vi "Y.vi"(8 "error in (no error)":errorcluster, 11 "MagSpec_Bella in":refnum<class "MagSpec_Bella.lvclass">) -> (0 "error out":errorcluster, 3 "MagSpec_Bella out":refnum<class "MagSpec_Bella.lvclass">)   [LabVIEW 2013, in "MagSpec_Bella.lvclass"]
uses:
  MagSpec_Bella.lvclass
  Controls/finalCalib--Cluster.ctl
  MagSpec_Bella.lvclass/MagSpec_Bella.ctl
  <vilib>/Analysis/1siggen.llb/Ramp Pattern by Delta.vi
  <vilib>/Analysis/NI_AALBase.lvlib
panel:
  out "Working":i32[](array[numeric])
  out "GOOD - not working":i32[](array[numeric])
  out "G":i32[](array[numeric])
  out "pixel angle (y)(pixel)":dbl[][](graph)
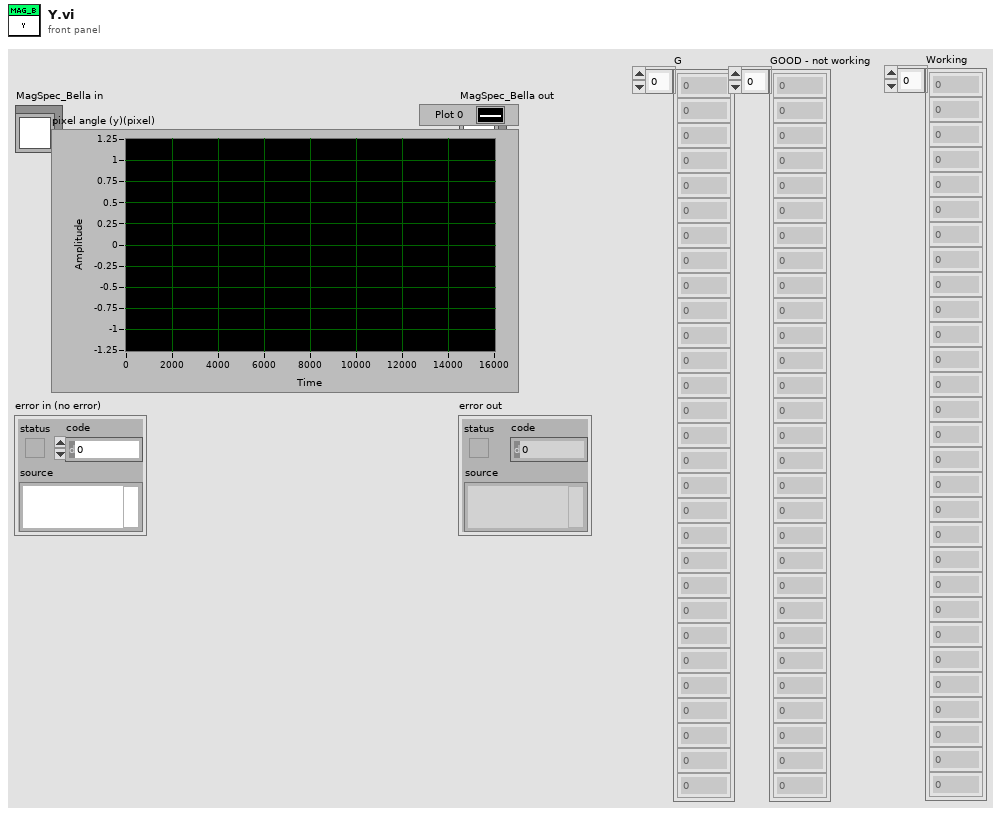
[diagram p1: front panel]
types:
  T1 = typedef "finalCalib--Cluster.ctl" = cluster{"X":dbl[][], "xi":dbl[][], "delta momentum":dbl, "Y":dbl[][], "yi":dbl[][], "angle (Y)":dbl[], "delta angle":dbl, "scale delta angle":dbl, "intraX":dbl, "intraY":dbl, "mask":dbl[][]}
  T2 = typedef "Calibration_Pixel_based.ctl" = cluster{"y1(pixel)":dbl[], "y2(pixel)":dbl[], "dp/B [MeV/C/B] (pixel)":dbl[], "energyDependence Input(pixel)":dbl[], "bending angle [deg](pixel)":dbl[], "total path(pixel)":dbl[], "pixel angle (y)(pixel)":dbl[], "energy dependence (pixel)":dbl[], "charge compensation (pixel)":dbl[], "Momentum [MeV/C](pixel)":dbl[], "angular compensation(pixel)":dbl[]}
  T3 = typedef "CameraSettings_File.ctl" = cluster{"FOV [mm]":dbl, "Left edge [mm]":dbl, "ROI Y offset":dbl, "ROI height":dbl, "ROI X offset":dbl, "ROI width":dbl, "Y center pixel":dbl, "Y Start":dbl, "Y End":dbl, "X Start":dbl, "X End":dbl, "rot [deg]":dbl}
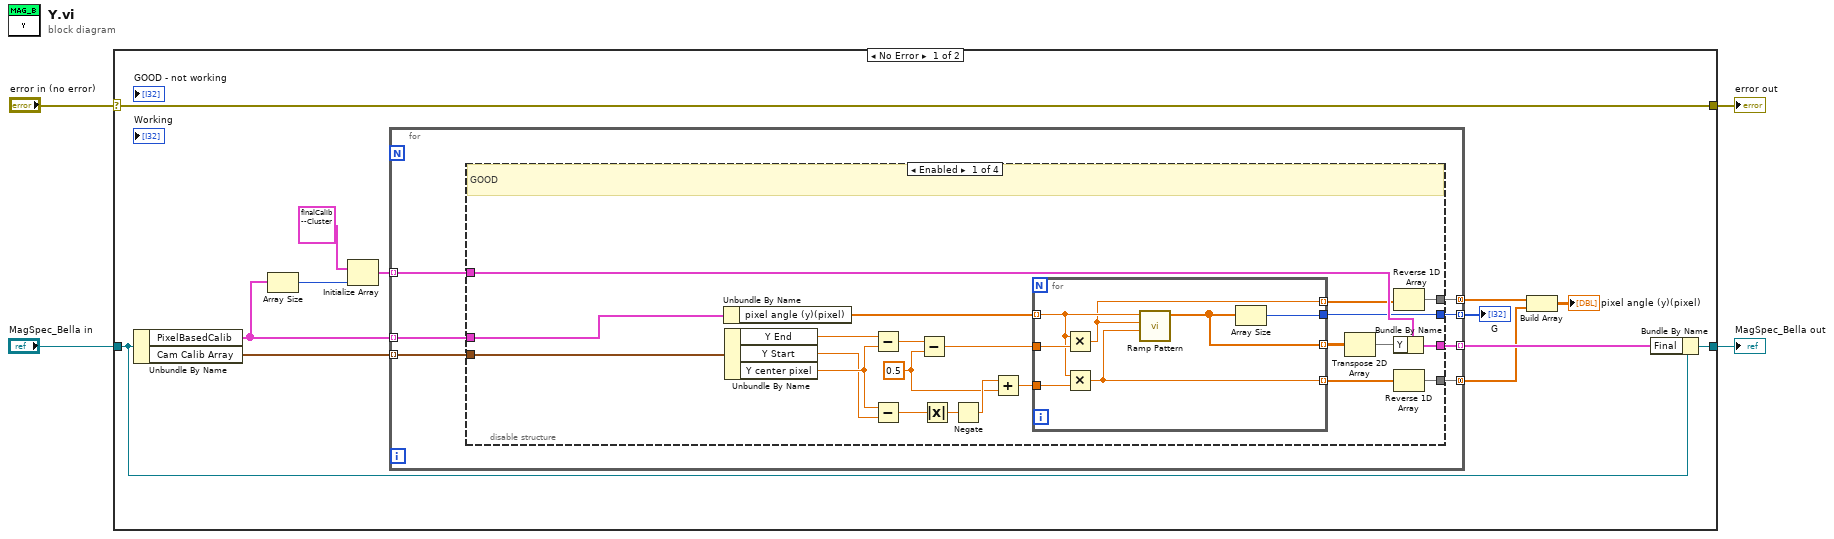
[diagram p0: block diagram]
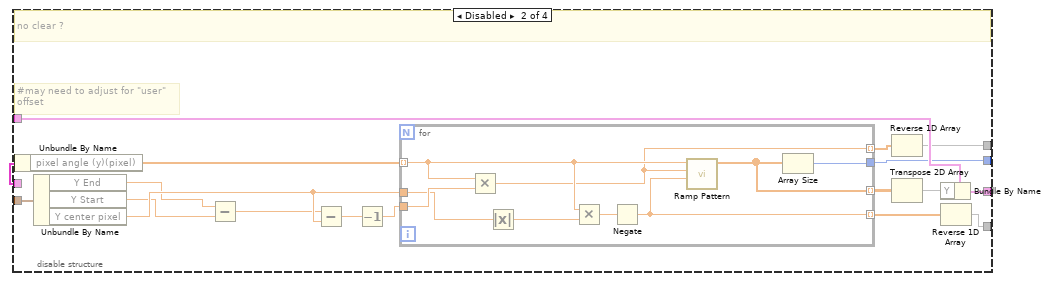
[diagram p2: hidden frame]
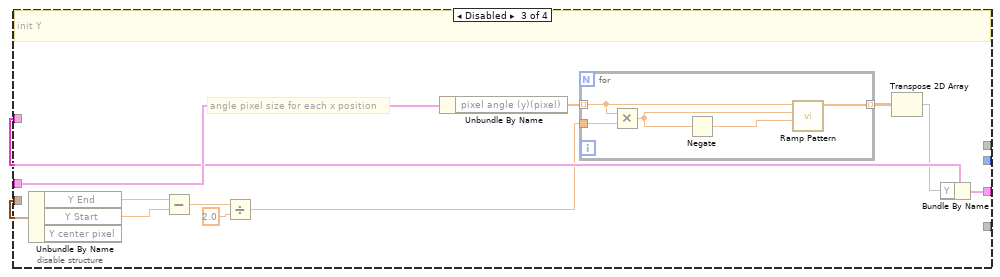
[diagram p3: hidden frame]
diagram:
  n1 = case shown="No Error" "error in (no error)" {
    selector: "error in (no error)" -> [w17 w99]
    tunnel: [w17 w99] -> w3
    tunnel: [w14 w98] -> w1
    tunnel: "MagSpec_Bella in" -> [w15 w98]
    frame No Error {
      n2 = Unbundle By Name(w15) -> ("PixelBasedCalib"=w9:T2[], "Cam Calib Array"=w10:T3[])
      n3 = Array Size(array=w9) -> (size(s)=w12:i32)
      n4 = Initialize Array(T1 {"X"=[], "xi"=[], "delta momentum"=0.0, "Y"=[], "yi"=[], "angle (Y)"=[], "delta angle"=0.0, "scale delta angle"=0.0, "intraX"=0.0, "intraY"=0.0, "mask"=[]} ("Cluster"), w12) -> (w11:T1[])
      n5 = for {
        tunnel: w9 -> [w24] mode=indexing
        tunnel: w11 -> [w23] mode=indexing
        tunnel: [w22] -> w16 mode=indexing
        tunnel: w10 -> [w21] mode=indexing
        tunnel: [w20] -> w8 mode=concatenating
        tunnel: [w19] -> w7 mode=concatenating
        tunnel: [w18] -> w5 mode=indexing
        n6 = disable-structure shown="Enabled" {
          disable-tunnel: w24 -> [w45 w70 w91 _]
          disable-tunnel: w23 -> [w44 w69 w89 _]
          disable-tunnel: [w42 w67 w87 _] -> w22
          disable-tunnel: w21 -> [w41 w66 w86 _]
          disable-tunnel: [w38 w59 _ _] -> w20
          disable-tunnel: [w37 w58 _ _] -> w19
          disable-tunnel: [w30 w54 _ _] -> w18
          frame Enabled {
            w26 = 0.5
            # "GOOD"
            n7 = Unbundle By Name(w45) -> ("pixel angle (y)(pixel)"=w39:dbl[])
            n8 = Unbundle By Name(w41) -> ("Y End"=w40:dbl, "Y Start"=w35:dbl, "Y center pixel"=w36:dbl)
            n9 = Subtract(x=w40, y=w36) -> (x-y=w29:dbl)
            n10 = Subtract(x=w36, y=w35) -> (x-y=w34:dbl)
            n11 = Subtract(x=w29, y=w26) -> (x-y=w28:dbl)
            n12 = Absolute Value(x=w34) -> (abs(x)=w33:dbl)
            n13 = Negate(x=w33) -> (-x=w27:dbl)
            n14 = Add(x=w27, y=w26) -> (x+y=w25:dbl)
            n15 = for {
              tunnel: w39 -> [w50] mode=indexing
              tunnel: [w53] -> w46 mode=indexing
              tunnel: w28 -> [w52]
              tunnel: w25 -> [w51]
              tunnel: [w49] -> w32 mode=indexing
              tunnel: [w48] -> w31 mode=indexing
              tunnel: [w47] -> w30
              n16 = Multiply(x=w50, y=w52) -> (x*y=w49:dbl)
              n17 = Multiply(x=w50, y=w51) -> (x*y=w48:dbl)
              n18 = call-poly <vilib>:"Ramp Pattern.vi"("start"=w48, "end"=w49, "delta"=w50) -> ("Ramp Pattern"=w53:dbl[])  [unwired: 6 in, 2 out]
              n19 = Array Size(array=w53) -> (size(s)=w47:i32)
            }
            n20 = Transpose 2D Array(2D array=w46) -> (transposed array=w43:dbl[][])
            n21 = Reverse 1D Array(array=w32) -> (reversed array=w37:dbl[])
            n22 = Bundle By Name(cluster=w44, "Y"=w43) -> (w42:T1)
            n23 = Reverse 1D Array(array=w31) -> (reversed array=w38:dbl[])
          }
          frame Disabled {
            # "#may need to adjust for \"user\"\noffset"
            # "no clear ?"
            n24 = Unbundle By Name(w70) -> ("pixel angle (y)(pixel)"=w62:dbl[])
            n25 = Unbundle By Name(w66) -> ("Y End"=w64:dbl, "Y Start"=w55:dbl, "Y center pixel"=w65:dbl)
            n26 = Subtract(x=w64, y=w55) -> (x-y=w63:dbl)
            n27 = Subtract(x=w63, y=w65) -> (x-y=w57:dbl)
            n28 = Decrement(x=w57) -> (x-1=w56:dbl)
            n29 = for {
              tunnel: w62 -> [w76] mode=indexing
              tunnel: [w73] -> w71 mode=indexing
              tunnel: w56 -> [w80]
              tunnel: w65 -> [w79]
              tunnel: [w75] -> w61 mode=indexing
              tunnel: [w74] -> w60 mode=indexing
              tunnel: [w72] -> w54
              n30 = Multiply(x=w76, y=w80) -> (x*y=w74:dbl)
              n31 = Absolute Value(x=w79) -> (abs(x)=w78:dbl)
              n32 = Multiply(x=w76, y=w78) -> (x*y=w77:dbl)
              n33 = Negate(x=w77) -> (-x=w75:dbl)
              n34 = call-poly <vilib>:"Ramp Pattern.vi"("start"=w75, "end"=w74, "delta"=w76) -> ("Ramp Pattern"=w73:dbl[])  [unwired: 6 in, 2 out]
              n35 = Array Size(array=w73) -> (size(s)=w72:i32)
            }
            n36 = Reverse 1D Array(array=w60) -> (reversed array=w58:dbl[])
            n37 = Transpose 2D Array(2D array=w71) -> (transposed array=w68:dbl[][])
            n38 = Bundle By Name(cluster=w69, "Y"=w68) -> (w67:T1)
            n39 = Reverse 1D Array(array=w61) -> (reversed array=w59:dbl[])
          }
          frame Disabled {
            # "angle pixel size for each x position"
            # "init Y"
            n40 = Unbundle By Name(w86) -> ("Y End"=w85:dbl, "Y Start"=w84:dbl)  [unwired: 1 out]
            n41 = Subtract(x=w85, y=w84) -> (x-y=w83:dbl)
            n42 = Divide(x=w83, y=2.0) -> (x/y=w81:dbl)
            n43 = Unbundle By Name(w91) -> ("pixel angle (y)(pixel)"=w90:dbl[])
            n44 = for {
              tunnel: w90 -> [w96] mode=indexing
              tunnel: [w97] -> w92 mode=indexing
              tunnel: w81 -> [w95]
              n45 = Multiply(x=w96, y=w95) -> (x*y=w93:dbl)
              n46 = Negate(x=w93) -> (-x=w94:dbl)
              n47 = call-poly <vilib>:"Ramp Pattern.vi"("start"=w94, "end"=w93, "delta"=w96) -> ("Ramp Pattern"=w97:dbl[])  [unwired: 6 in, 2 out]
            }
            n48 = Transpose 2D Array(2D array=w92) -> (transposed array=w88:dbl[][])
            n49 = Bundle By Name(cluster=w89, "Y"=w88) -> (w87:T1)
          }
          frame Disabled {
          }
        }
      }
      "G" <- w5
      n50 = Build Array(w7, w8) -> (→"pixel angle (y)(pixel)":dbl[][])
      n51 = Bundle By Name(cluster=w15, "Final"=w16) -> (w14:refnum<class "MagSpec_Bella.lvclass">)
    }
    frame Error {
    }
  }
  "error out" <- w3
  "MagSpec_Bella out" <- w1
